vi "Agilent PNA Config1.vi"(0 "VISA session":refnum<visa-resource-name>="GPIB0::16::INSTR", 5 "Start Freq (10.0 E+6)":dbl=1000000000.0 format="%.2p", 7 "Stop Freq (26.4 E+9)":dbl=10000000000.0 format="%.2p", 9 "Sweep Points (801)":i32=201, 11 "Measurement Type (0: S11)":i32(ring) items=["S11", "S12", "S21", "S22", "A", "B", "R1", "R2", "A/B", "B/A"], 14 "Bandwidth (1000.0)":dbl=1000.0 format="%.2p") -> (4 "dup VISA session":refnum<visa-resource-name>="GPIB0::16::INSTR", 10 "Sweep Time":dbl=0.74811474 format="%.2p")   [LabVIEW 2018]
doc: "This VI configures the sweep parameters and reads data from the analyzer.\n\nNote: To see the data on the analyzer after running the program, from the front panel click: Trace - Math/Memory - Memory Trace"
uses:
  Agilent PNA Series/Agilent PNA Series.lvlib
panel:
  in  "CW Points":dbl=100.0
  in  "Trigger Mode (1: Continuous)":u16(ring)=2 items=["Hold", "Continuous", "Count"]
  in  "Smooth Aperture (25.0)":dbl=25.0 format="%.2p"
  in  "Smooth State":bool
  in  "CW Frq.":dbl=1000000000.0
  in  "Power Level":dbl=-10.0
  in  "Sweep Type":string(combo)="LINear"
  in  "AVG Factor":i32=5
  in  "Average?":bool
  in  "Autoscale?":bool
  in  "Format":string(combo)="MLOGarithmic"
  in  "Measurement Name (MY_MEAS)":string="MY_MEAS"
  # "(c) 2005-2015 National Instruments.  ALL RIGHTS RESERVED."
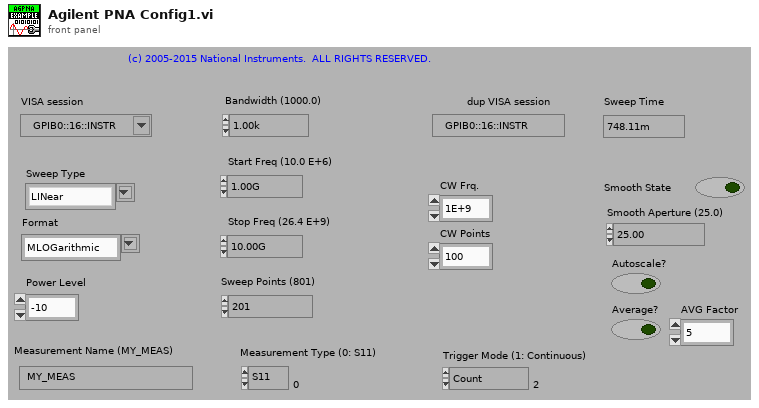
[diagram p1: front panel]
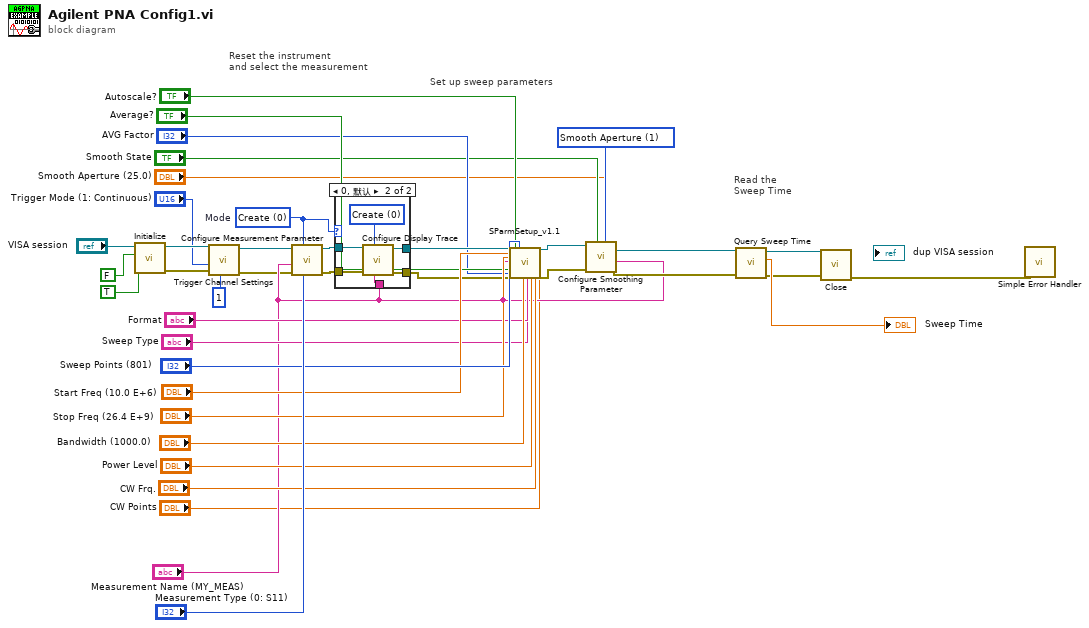
[diagram p0: block diagram]
diagram:
  w11 = u16 1 items=["Smooth Points", "Smooth Aperture"] ("Mode (0: Smooth Points)")
  w32 = u16 0 items=["Create", "Delete", "Select"]  # Mode
  # "Read the \nSweep Time"
  # "Set up sweep parameters"
  # "Reset the instrument\nand select the measurement"
  n1 = call "Initialize.vi"("Reset (T: Reset)"=TRUE, "ID Query (T: Check)"=FALSE, "Instrument Resource Name"="VISA session") -> ("error out"=w8:errorcluster, "dup VISA session"=w9:refnum<visa-resource-name>)  [unwired: 7 in]
  n2 = call "Trigger Channel Settings.vi"("Trigger Count (1)"=1, "Error In (no error)"=w8, "Trigger Mode (1: Continuous)"="Trigger Mode (1: Continuous)", "VISA session"=w9) -> ("Error Out"=w7:errorcluster, "dup VISA session"=w6:refnum<visa-resource-name>)  [unwired: 6 in]
  n3 = call "Configure Measurement Parameter.vi"("Measurement Type (0: S11)"="Measurement Type (0: S11)", "Mode (0: Create)"=w32, "Error In (no error)"=w7, "Measurement Name (MY_MEAS)"="Measurement Name (MY_MEAS)", "VISA Resource Name"=w6) -> ("Error Out"=w33:errorcluster, "VISA Resource Name Out"=w34:refnum<visa-resource-name>)  [unwired: 5 in]
  n4 = case shown="0, 默认" w32 {
    tunnel: w34 -> [w41 w47]
    tunnel: [w41 w46] -> w25
    tunnel: w33 -> [w40 w45]
    tunnel: [w40 w44] -> w26
    tunnel: "Measurement Name (MY_MEAS)" -> [_ w42]
    frame 2 {
    }
    frame 0, Default {
      w43 = u16 0 items=["Create", "Delete"] ("Mode (0: Create)")
      n5 = call "Configure Display Trace.vi"("Measurement Name (MY_MEAS)"=w42, "Mode (0: Create)"=w43, "Error In (no error)"=w45, "VISA Resource Name"=w47) -> ("Error Out"=w44:errorcluster, "VISA Resource Name Out"=w46:refnum<visa-resource-name>)  [unwired: 6 in]
    }
  }
  n6 = call "SParmSetup_v1.1.vi"("VISA IN"=w25, "Start Frequency"="Start Freq (10.0 E+6)", "Stop Frequency"="Stop Freq (26.4 E+9)", "Filename"="Measurement Name (MY_MEAS)", "Average?"="Average?", "AVG Factor"="AVG Factor", "error in"=w26, "Autoscale?"="Autoscale?", "Points"="Sweep Points (801)", "IF BW"="Bandwidth (1000.0)", "Format"="Format", "Sweep Type"="Sweep Type", "Power Level"="Power Level", "CW Frq."="CW Frq.", "CW Points"="CW Points") -> ("VISA Out"=w17:refnum<visa-resource-name>, "error out"=w15:errorcluster)  [unwired: 11 in]
  n7 = call "Configure Smoothing Parameter.vi"("Smooth Aperture (25.0)"="Smooth Aperture (25.0)", "Mode (0: Smooth Points)"=w11, "Smooth State (F: Off)"="Smooth State", "Error In (no error)"=w15, "Measurement Name (MY_MEAS)"="Measurement Name (MY_MEAS)", "VISA Resource Name"=w17) -> ("Error Out"=w14:errorcluster, "VISA Resource Name Out"=w16:refnum<visa-resource-name>)  [unwired: 4 in]
  n8 = call "Query Sweep Time.vi"("Error In (no error)"=w14, "VISA Resource Name"=w16) -> ("Error Out"=w1:errorcluster, "Sweep Time"=→"Sweep Time":dbl, "VISA Resource Name Out"=w2:refnum<visa-resource-name>)  [unwired: 7 in]
  n9 = call "Close.vi"("Error In (no error)"=w1, "VISA Resource Name"=w2) -> ("Error Out"=w37:errorcluster)  [unwired: 9 in]
  n10 = call <vilib>:"Simple Error Handler.vi"("error in (no error)"=w37) -> ()  [unwired: 4 in, 5 out]
